vi "04_MCLB.vi"() -> ()   [LabVIEW 2020]
uses:
  9dc58315-b66f-4daf-a33c-5342c64e7d45.vi
panel:
  in  "Multicolumn Listbox":i32(listbox)
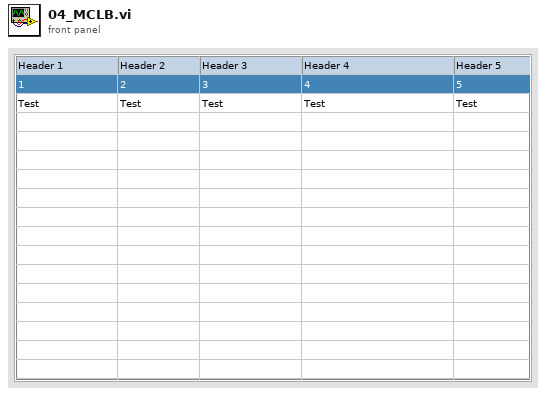
[diagram p1: front panel]
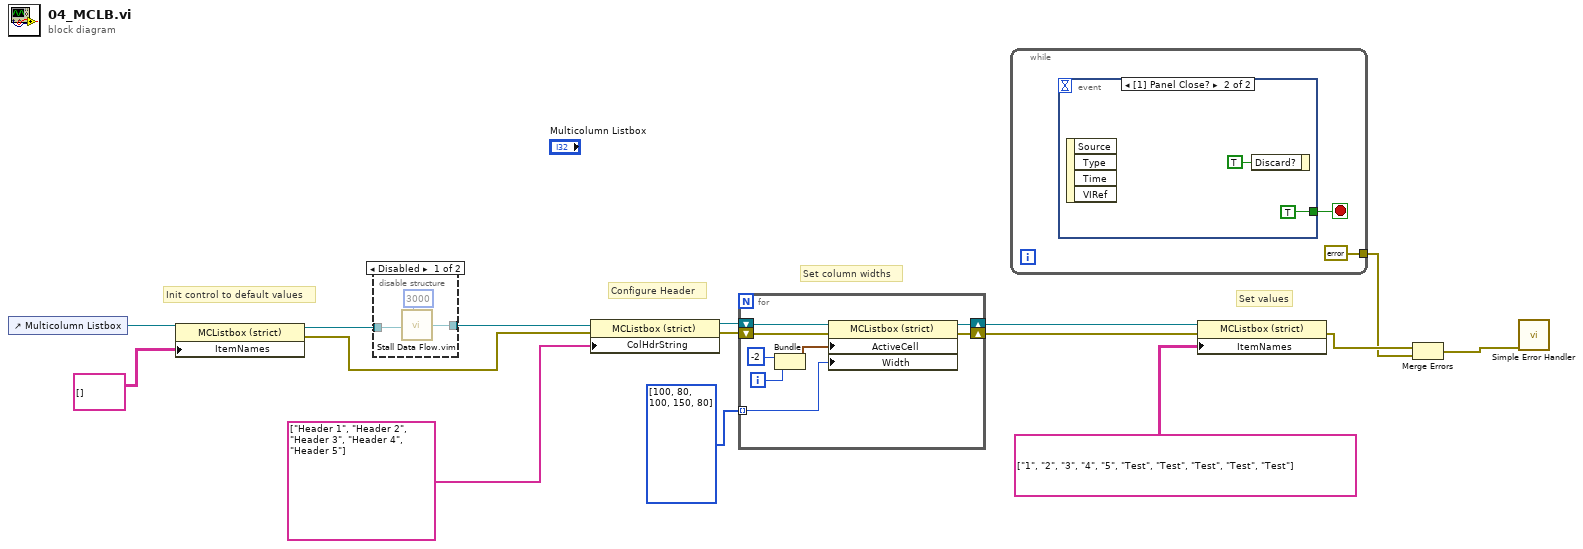
[diagram p0: block diagram]
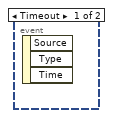
[diagram p2: hidden frame]
diagram:
  # "Set column widths"
  # "Set values"
  # "Configure Header"
  # "Init control to default values"
  n1 = control-ref of="Multicolumn Listbox"() -> (w8:refnum<vi>)
  n2 = property class="MCListbox (strict)"(reference=w8, "ItemNames"=string[][] [] ("Item Names")) -> (reference out=w11:refnum<vi>, error out=w10:errorcluster)  [unwired: 1 in]
  n3 = disable-structure shown="Disabled" {
    disable-tunnel: [w18 w19] -> w12
    disable-tunnel: w11 -> [w16 w19]
    frame Disabled {
      n4 = call "Stall Data Flow.vim"("value in"=w16, "milliseconds to wait"=u32 3000) -> ("value out"=w18:refnum<vi>)  [unwired: 1 out]
    }
    frame Enabled {
    }
  }
  n5 = property class="MCListbox (strict)"(reference=w12, error in=w10, "ColHdrString"=string[] ["Header 1", "Header 2", "Header 3", "Header 4", "Header 5"] ("Column Header Strings[]")) -> (reference out=w7:refnum<vi>, error out=w5:errorcluster)
  n6 = for {
    shift-right: [w26] -> w6
    shift-left: w7 -> [w27]
    shift-right: [w24] -> w4
    shift-left: w5 -> [w25]
    tunnel: i32[] [100, 80, 100, 150, 80] ("Column Sizes[]") -> [w20] mode=indexing
    i -> [w22]
    n7 = Bundle(-2, w22) -> (w23:cluster{i32, i32})  [unwired: 1 in]
    n8 = property class="MCListbox (strict)"(reference=w27, error in=w25, "ActiveCell"=w23, "Width"=w20) -> (reference out=w26:refnum<vi>, error out=w24:errorcluster)
  }
  n9 = while {
    tunnel: [errorcluster {"status"=FALSE, "code"=0, "source"=""} ("error constant")] -> w1
    stop <- w29 stop-if-true
    n10 = event shown="[1] Panel Close?" {
      selector: _ -> [_ _]
      dyn-events: _ -> [_ _]
      timeout: _ -> [_ _]
      tunnel: [_ TRUE] -> w29
      event Timeout {
        n11 = event-data() -> ()  [unwired: 1 in, 3 out]
      }
      event Panel Close? {
        n12 = event-data() -> ()  [unwired: 1 in, 4 out]
        n13 = event-data("Discard?"=TRUE) -> ()  [unwired: 1 in, 1 out]
      }
    }
  }
  n14 = property class="MCListbox (strict)"(reference=w6, error in=w4, "ItemNames"=string[][] [["1", "2", "3", "4", "5"], ["Test", "Test", "Test", "Test", "Test"]] ("Item Names")) -> (error out=w14:errorcluster)  [unwired: 1 out]
  n15 = Merge Errors(w14, w1) -> (w2:errorcluster)
  n16 = call <vilib>:"Simple Error Handler.vi"("error in (no error)"=w2) -> ()  [unwired: 4 in, 5 out]
